vi "PickupTool Class Sandbox.vi"() -> ()   [LabVIEW 2011]
uses:
  PickupTool Class.lvclass
panel:
  out "error out":errorcluster
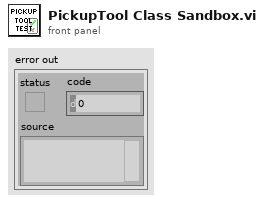
[diagram p1: front panel]
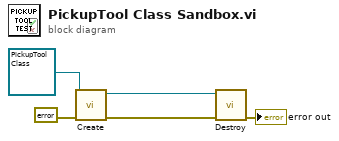
[diagram p0: block diagram]
diagram:
  n1 = call-dynamic "Create.vi"("error in (no error)"=errorcluster {"status"=FALSE, "code"=0, "source"=""} ("error constant"), "PickupTool Class in"=refnum<class "PickupTool Class.lvclass"> refnum) -> ("error out"=w4:errorcluster, "PickupTool Class out"=w5:refnum<class "PickupTool Class.lvclass">)  [unwired: 8 in]
  n2 = call-dynamic "Destroy.vi"("error in (no error)"=w4, "PickupTool Class in"=w5) -> ("error out"=→"error out":errorcluster)  [unwired: 8 in, 1 out]
